vi "OE1022D_Query PLL&Overload.vi"(6 "Timeout":u32=1000, 8 "Error in (no error)":errorcluster caption="error out（no error）", 9 "Remote Mode":u16(ring) items=["USB", "RS232", "GPIB"], 10 "Channel":u16(ring)=1 items=["A"=1, "B"=2], 11 "VISA resource name":refnum<visa-resource-name>) -> (0 "Error out":errorcluster caption="error out", 1 "Output String":string, 2 "OE1022D_Query PLL&Overload":T1, 3 "VISA resource  out":refnum<visa-resource-name>)   [LabVIEW 2019]
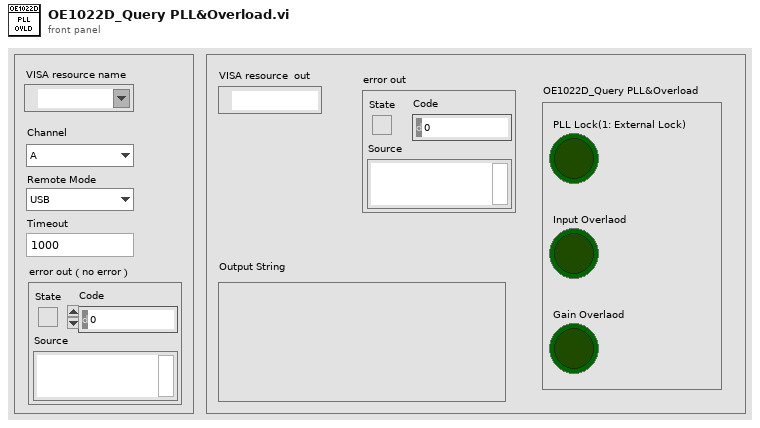
[diagram p1: front panel]
types:
  T1 = cluster{"PLL Lock(1: External Lock)":bool, "Input Overlaod":bool, "Gain Overlaod":bool}
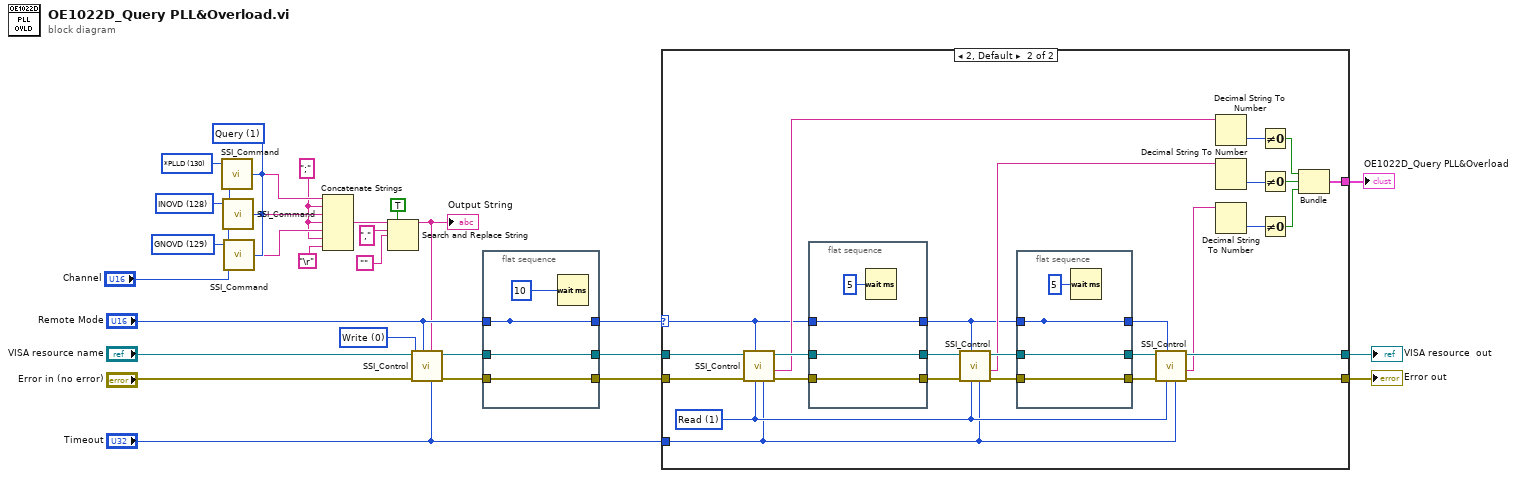
[diagram p0: block diagram]
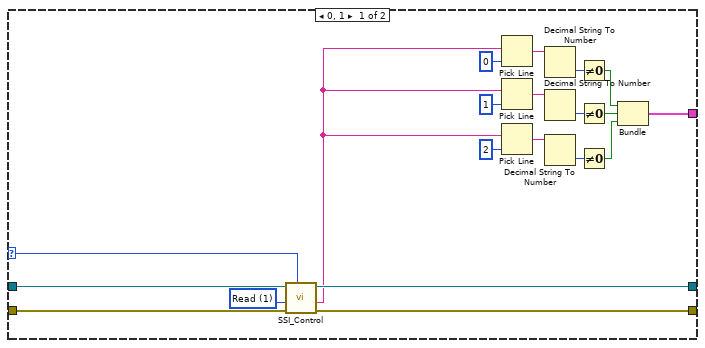
[diagram p2: hidden frame]
diagram:
  w12 = u16 129 items=["ISRC", "IGND", "ICPL", "ILIN", "PHAS", "FMOD", "RSLP", "FREQ", "SWPT", "SLLM", "SULM", "SSLL", "SSLG", "STLM", "SWRM", "IRNG", "SENS", "RMOD", "OFLT", "OFSL", "SYNC", "DMOD", "HARM", "DARB", "SWVT", "SLVL", "SVLL", "SVUL", "SVSL", "SVSG", "SVTM", "SVRM", "RALL", "SNAP", "OUTP", "OAUX", "COUT", "CAUX", "COFP", "CEXP", "FPOP", "OEXP", "*IDN", "*RST", "OVLD", "INOV", "GNOV", "*PLL", "SSET", "RSET", "AGAN", "APHS", "ARSV", "ASCL", "EQCD", "EQCS", "SPED", "SRAT", "SLEN", "SSLE", "STRG", "SPRM", "STRD", "PAUS", "REST", "SPTS", "TRCA", "TEMP", "RSTU", "IHNZ", "DEQU", "SADD", "ARNG", "CSPE", "ISRCD", "IGNDD", "ICPLD", "ILIND", "PHASD", "FMODD", "RSLPD", "FREQD", "SWPTD", "SLLMD", "SULMD", "SSLLD", "SSLGD", "STLMD", "SWRMD", "SENSD", "RMODD", "OFLTD", "OFSLD", "SYNCD", "HARMD", "EQCDD", "EQCSD", "SNAPD", "OUTPD", "SWVTD", "SLVLD", "SVLLD", "SVULD", "SVSLD", "SVSGD", "SVTMD", "SVRMD", "SVDCD", "ARSVD", "AGAND", "APHSD", "ASCLD", "FPOPD", "CAUXD", "OEXPD", "SPEDD", "SRATD", "SLEND", "SSLED", "STRGD", "SPRMD", "STRDD", "PAUSD", "RESTD", "SPTSD", "TRCAD", "*IDND", "*RSTD", "INOVD", "GNOVD", "*PLLD", "SSETD", "RSETD", "RALLD"] ("Command Type")
  w13 = u16 128 items=["ISRC", "IGND", "ICPL", "ILIN", "PHAS", "FMOD", "RSLP", "FREQ", "SWPT", "SLLM", "SULM", "SSLL", "SSLG", "STLM", "SWRM", "IRNG", "SENS", "RMOD", "OFLT", "OFSL", "SYNC", "DMOD", "HARM", "DARB", "SWVT", "SLVL", "SVLL", "SVUL", "SVSL", "SVSG", "SVTM", "SVRM", "RALL", "SNAP", "OUTP", "OAUX", "COUT", "CAUX", "COFP", "CEXP", "FPOP", "OEXP", "*IDN", "*RST", "OVLD", "INOV", "GNOV", "*PLL", "SSET", "RSET", "AGAN", "APHS", "ARSV", "ASCL", "EQCD", "EQCS", "SPED", "SRAT", "SLEN", "SSLE", "STRG", "SPRM", "STRD", "PAUS", "REST", "SPTS", "TRCA", "TEMP", "RSTU", "IHNZ", "DEQU", "SADD", "ARNG", "CSPE", "ISRCD", "IGNDD", "ICPLD", "ILIND", "PHASD", "FMODD", "RSLPD", "FREQD", "SWPTD", "SLLMD", "SULMD", "SSLLD", "SSLGD", "STLMD", "SWRMD", "SENSD", "RMODD", "OFLTD", "OFSLD", "SYNCD", "HARMD", "EQCDD", "EQCSD", "SNAPD", "OUTPD", "SWVTD", "SLVLD", "SVLLD", "SVULD", "SVSLD", "SVSGD", "SVTMD", "SVRMD", "SVDCD", "ARSVD", "AGAND", "APHSD", "ASCLD", "FPOPD", "CAUXD", "OEXPD", "SPEDD", "SRATD", "SLEND", "SSLED", "STRGD", "SPRMD", "STRDD", "PAUSD", "RESTD", "SPTSD", "TRCAD", "*IDND", "*RSTD", "INOVD", "GNOVD", "*PLLD", "SSETD", "RSETD", "RALLD"] ("Command Type")
  w14 = u16 130 items=["ISRC", "IGND", "ICPL", "ILIN", "PHAS", "FMOD", "RSLP", "FREQ", "SWPT", "SLLM", "SULM", "SSLL", "SSLG", "STLM", "SWRM", "IRNG", "SENS", "RMOD", "OFLT", "OFSL", "SYNC", "DMOD", "HARM", "DARB", "SWVT", "SLVL", "SVLL", "SVUL", "SVSL", "SVSG", "SVTM", "SVRM", "RALL", "SNAP", "OUTP", "OAUX", "COUT", "CAUX", "COFP", "CEXP", "FPOP", "OEXP", "*IDN", "*RST", "OVLD", "INOV", "GNOV", "*PLL", "SSET", "RSET", "AGAN", "APHS", "ARSV", "ASCL", "EQCD", "EQCS", "SPED", "SRAT", "SLEN", "SSLE", "STRG", "SPRM", "STRD", "PAUS", "REST", "SPTS", "TRCA", "TEMP", "RSTU", "IHNZ", "DEQU", "SADD", "ARNG", "CSPE", "ISRCD", "IGNDD", "ICPLD", "ILIND", "PHASD", "FMODD", "RSLPD", "FREQD", "SWPTD", "SLLMD", "SULMD", "SSLLD", "SSLGD", "STLMD", "SWRMD", "SENSD", "RMODD", "OFLTD", "OFSLD", "SYNCD", "HARMD", "EQCDD", "EQCSD", "SNAPD", "OUTPD", "SWVTD", "SLVLD", "SVLLD", "SVULD", "SVSLD", "SVSGD", "SVTMD", "SVRMD", "SVDCD", "ARSVD", "AGAND", "APHSD", "ASCLD", "FPOPD", "CAUXD", "OEXPD", "SPEDD", "SRATD", "SLEND", "SSLED", "STRGD", "SPRMD", "STRDD", "PAUSD", "RESTD", "SPTSD", "TRCAD", "*IDND", "*RSTD", "INOVD", "GNOVD", "*PLLD", "SSETD", "RSETD", "RALLD"] ("Command Type")
  w16 = ";"
  w20 = u16 1 items=["Set", "Query"] ("Opera")
  w27 = u16 0 items=["Write", "Read"] ("Control")
  n1 = call "SSI_Command.vi"("Opera"=w20, "channel"="Channel", "Command Type"=w14) -> ("Output string"=w19:string)  [unwired: 1 in]
  n2 = call "SSI_Command.vi"("Opera"=w20, "channel"="Channel", "Command Type"=w13) -> ("Output string"=w18:string)  [unwired: 1 in]
  n3 = call "SSI_Command.vi"("Opera"=w20, "channel"="Channel", "Command Type"=w12) -> ("Output string"=w17:string)  [unwired: 1 in]
  n4 = Concatenate Strings(w19, w16, w18, w16, w17, w16, "\r") -> (w10:string)
  n5 = Search and Replace String(replace all?=TRUE ("替换全部？(F)"), input string=w10, search string="," ("搜索字符串"), replace string="") -> (result string=w9:string)  [unwired: 4 in, 3 out]
  "Output String" <- w9
  n6 = call "SSI_Control.vi"("Tineout"="Timeout", "Write Buffer"=w9, "Remote Mode"="Remote Mode", "Error in (no error)"="Error in (no error)", "Control"=w27, "VISA resource name"="VISA resource name") -> ("Error out"=w25:errorcluster, "VISA resource  out"=w24:refnum<visa-resource-name>)  [unwired: 2 in, 2 out]
  n7 = flat-sequence {
    tunnel: [w32] -> w23
    tunnel: w25 -> [w32]
    tunnel: [w31] -> w22
    tunnel: w24 -> [w31]
    tunnel: "Remote Mode" -> [w30]
    tunnel: [w30] -> _
    tunnel: [w30] -> w5
    frame #0 {
      n8 = Wait (ms)(milliseconds to wait=u32 10 ("等待时间（毫秒）")) -> ()  [unwired: 1 out]
    }
  }
  n9 = case shown="2, Default" w5 {
    selector: w5 -> [w34 w56]
    tunnel: w23 -> [w38 w79]
    tunnel: w22 -> [w39 w78]
    tunnel: [w40 w74] -> w3
    tunnel: [w36 w65] -> w2
    tunnel: [w37 w64] -> w1
    tunnel: "Timeout" -> [_ w53]
    frame 0, 1 {
      w35 = u16 1 items=["Write", "Read"] ("Control")
      n10 = call "SSI_Control.vi"("Remote Mode"=w34, "Error in (no error)"=w38, "Control"=w35, "VISA resource name"=w39) -> ("Error out"=w36:errorcluster, "Read Buffer"=w33:string, "VISA resource  out"=w37:refnum<visa-resource-name>)  [unwired: 4 in, 1 out]
      n11 = Pick Line(multi-line string=w33, line index=0 ("行索引")) -> (output string=w50:string)  [unwired: 1 in]
      n12 = Pick Line(multi-line string=w33, line index=1 ("行索引")) -> (output string=w51:string)  [unwired: 1 in]
      n13 = Pick Line(multi-line string=w33, line index=2 ("行索引")) -> (output string=w46:string)  [unwired: 1 in]
      n14 = Decimal String To Number(string=w50) -> (number=w41:i32)  [unwired: 2 in, 1 out]
      n15 = Decimal String To Number(string=w51) -> (number=w42:i32)  [unwired: 2 in, 1 out]
      n16 = Decimal String To Number(string=w46) -> (number=w43:i32)  [unwired: 2 in, 1 out]
      n17 = Not Equal To 0?(x=w41) -> (x != 0?=w49:bool)
      n18 = Not Equal To 0?(x=w42) -> (x != 0?=w52:bool)
      n19 = Not Equal To 0?(x=w43) -> (x != 0?=w44:bool)
      n20 = Bundle(w49, w52, w44) -> (w40:cluster{bool, bool, bool})  [unwired: 1 in]
    }
    frame 2, Default {
      w63 = u16 1 items=["Write", "Read"] ("Control")
      n21 = call "SSI_Control.vi"("Tineout"=w53, "Remote Mode"=w56, "Error in (no error)"=w79, "Control"=w63, "VISA resource name"=w78) -> ("Error out"=w73:errorcluster, "Read Buffer"=w60:string, "VISA resource  out"=w72:refnum<visa-resource-name>)  [unwired: 3 in, 1 out]
      n22 = flat-sequence {
        tunnel: [w87] -> w71
        tunnel: w73 -> [w87]
        tunnel: [w86] -> w70
        tunnel: w72 -> [w86]
        tunnel: w56 -> [w84]
        tunnel: [w84] -> w55
        frame #0 {
          n23 = Wait (ms)(milliseconds to wait=u32 5 ("等待时间（毫秒）")) -> ()  [unwired: 1 out]
        }
      }
      n24 = call "SSI_Control.vi"("Tineout"=w53, "Remote Mode"=w55, "Error in (no error)"=w71, "Control"=w63, "VISA resource name"=w70) -> ("Error out"=w68:errorcluster, "Read Buffer"=w59:string, "VISA resource  out"=w69:refnum<visa-resource-name>)  [unwired: 3 in, 1 out]
      n25 = flat-sequence {
        tunnel: [w83] -> w67
        tunnel: w68 -> [w83]
        tunnel: [w82] -> w66
        tunnel: w69 -> [w82]
        tunnel: w55 -> [w80]
        tunnel: [w80] -> _
        tunnel: [w80] -> w54
        frame #0 {
          n26 = Wait (ms)(milliseconds to wait=u32 5 ("等待时间（毫秒）")) -> ()  [unwired: 1 out]
        }
      }
      n27 = call "SSI_Control.vi"("Tineout"=w53, "Remote Mode"=w54, "Error in (no error)"=w67, "Control"=w63, "VISA resource name"=w66) -> ("Error out"=w65:errorcluster, "Read Buffer"=w62:string, "VISA resource  out"=w64:refnum<visa-resource-name>)  [unwired: 3 in, 1 out]
      n28 = Decimal String To Number(string=w60) -> (number=w57:i32)  [unwired: 2 in, 1 out]
      n29 = Decimal String To Number(string=w59) -> (number=w58:i32)  [unwired: 2 in, 1 out]
      n30 = Decimal String To Number(string=w62) -> (number=w61:i32)  [unwired: 2 in, 1 out]
      n31 = Not Equal To 0?(x=w57) -> (x != 0?=w76:bool)
      n32 = Not Equal To 0?(x=w58) -> (x != 0?=w77:bool)
      n33 = Not Equal To 0?(x=w61) -> (x != 0?=w75:bool)
      n34 = Bundle(w76, w77, w75) -> (w74:cluster{bool, bool, bool})  [unwired: 1 in]
    }
  }
  "Error out" <- w2
  "VISA resource  out" <- w1
  "OE1022D_Query PLL&Overload" <- w3
